vi "CHAT_1.vi"() -> ()   [LabVIEW 2016]
panel:
  in  "ARRAY3":dbl[](array[numeric])
  out "Numeric Control_2":dbl
  out "Boolean_2":bool
  in  "Numeric Control_1":dbl
  in  "Boolean_1":bool
  in  "Stop Button":bool
  out "Usuario 2":string
  in  "Usuario 1":string
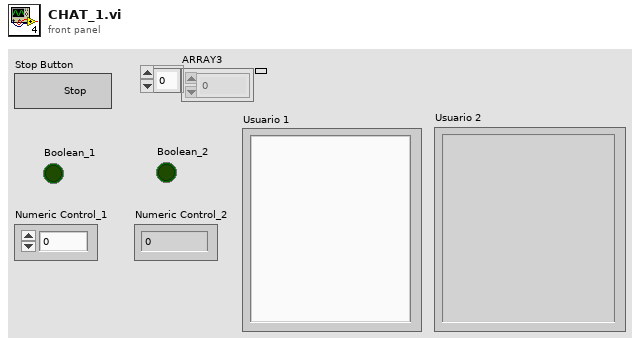
[diagram p1: front panel]
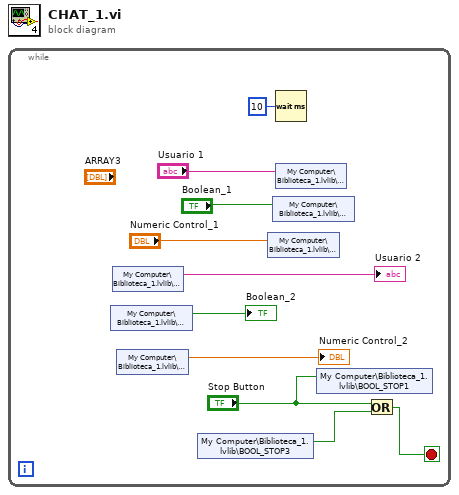
[diagram p0: block diagram]
diagram:
  n1 = while {
    stop <- w10 stop-if-true
    n2 = shared-variable "My Computer\\Biblioteca_1.lvlib\\BOOL3"() -> (→"Boolean_2":bool)  [unwired: 1 in, 1 out]
    n3 = shared-variable "My Computer\\Biblioteca_1.lvlib\\STR3"() -> (→"Usuario 2":string)  [unwired: 1 in, 1 out]
    n4 = shared-variable "My Computer\\Biblioteca_1.lvlib\\DBL3"() -> (→"Numeric Control_2":dbl)  [unwired: 1 in, 1 out]
    n5 = shared-variable "My Computer\\Biblioteca_1.lvlib\\BOOL_STOP3"() -> (w2:bool)  [unwired: 1 in, 1 out]
    n6 = shared-variable "My Computer\\Biblioteca_1.lvlib\\DBL1"("Numeric Control_1") -> ()  [unwired: 1 in, 1 out]
    n7 = shared-variable "My Computer\\Biblioteca_1.lvlib\\BOOL1"("Boolean_1") -> ()  [unwired: 1 in, 1 out]
    n8 = Wait (ms)(milliseconds to wait=u32 10) -> ()  [unwired: 1 out]
    n9 = shared-variable "My Computer\\Biblioteca_1.lvlib\\STR1"("Usuario 1") -> ()  [unwired: 1 in, 1 out]
    n10 = shared-variable "My Computer\\Biblioteca_1.lvlib\\BOOL_STOP1"("Stop Button") -> ()  [unwired: 1 in, 1 out]
    n11 = Or(x="Stop Button", y=w2) -> (x .or. y?=w10:bool)
  }
